vi "Actor Core.vi"(8 "error in":errorcluster, 11 "SensorCharm in":refnum<class "TimerSensorCharm.lvclass">) -> (0 "error out":errorcluster, 3 "Actor out":refnum<class "Actor.lvclass">)   [LabVIEW 2012, in "TimerSensor.lvlib" / "TimerSensorCharm.lvclass"]
doc: "(<B>Filename</B>: Actor Framework.lvlib:Actor.lvclass:Actor Core.vi)\n\nReceives messages to the actor, reacts to them, and initiates any error handling that may shut the actor down.\n\nDescendant classes may override this VI to append parallel tasks for the actor to complete while it handles messages. Overrides use the Call Parent Method node."
uses:
  TimerSensorCharm.lvclass
  <vilib>/ActorFramework/Actor/Actor.lvclass
  TimerView Sensor/Timer Direction.ctl
  Sensor Definition/SensorCharm.lvclass
  TimerSensorConfig.lvclass
  <vilib>/ActorFramework/Actor/Actor.lvclass/Actor.ctl
  <vilib>/ActorFramework/Message Enqueuer/Message Enqueuer.lvclass/Message Enqueuer.ctl
  Win8uiFramework/ViewableActor.lvclass/ViewableActor.ctl
  Sensor Definition/SensorCharm.lvclass/SensorCharm.ctl
  Sensor Definition/SensorInfo.lvclass/SensorInfo.ctl
  TimerSensorConfig.lvclass/TimerSensorConfig.ctl
  Sensor Messages/Update Sensor Info and Re-broadcast Msg/Update Sensor Info and Re-broadcast Msg.lvclass/Update Sensor Info and Re-broadcast Msg.ctl
  TimerView Sensor/Write Target Time.vi
  TimerView Sensor/Write Timer Direction.vi
  Sensor Definition/SensorInfo/Write Name.vi
  Sensor Definition/Write Description.vi
  Sensor Definition/SensorInfo/Write Config.vi
  Sensor Definition/SensorInfo/Write Sample Time.vi
  Win8uiFramework/Read Stop Event.vi
  Sensor Definition/SensorCharm/Read SensorInfo.vi
  Sensor Definition/SensorInfo/Read Name.vi
  Sensor Definition/SensorInfo/Read Description.vi
  Sensor Definition/Read Config.vi
  Sensor Definition/SensorInfo/Read Sample Time.vi
  TimerSensorConfig/Read Target Time.vi
  TimerSensorConfig/Read Timer Direction.vi
  <vilib>/ActorFramework/Message Enqueuer/Init from Existing Queue.vi
  <vilib>/ActorFramework/Message Enqueuer/Enqueue.vi
  <vilib>/ActorFramework/Message Priority Queue/Priority Enqueue.vi
  <vilib>/ActorFramework/Message Enqueuer/Message Enqueuer.lvclass
  Sensor Definition/SensorInfo.lvclass
  Sensor Definition/SensorConfig.lvclass
  Sensor Messages/Update Sensor Info and Re-broadcast Msg/Update Sensor Info and Re-broadcast Msg.lvclass
  Win8uiFramework/ViewableActor.lvclass
  TimerSensor.lvlib
panel:
  in  "Timer Direction":u16(ring) items=["Up", "Down"]
  in  "Timer Direction Enum":T1
  in  "Target Time":timestamp
  in  "Name":string="Name"
  in  "Sample Period (s)":dbl=1.0
  in  "Description":string="Description of what and/or where this sensor is."
  out "Title":string="Settings"
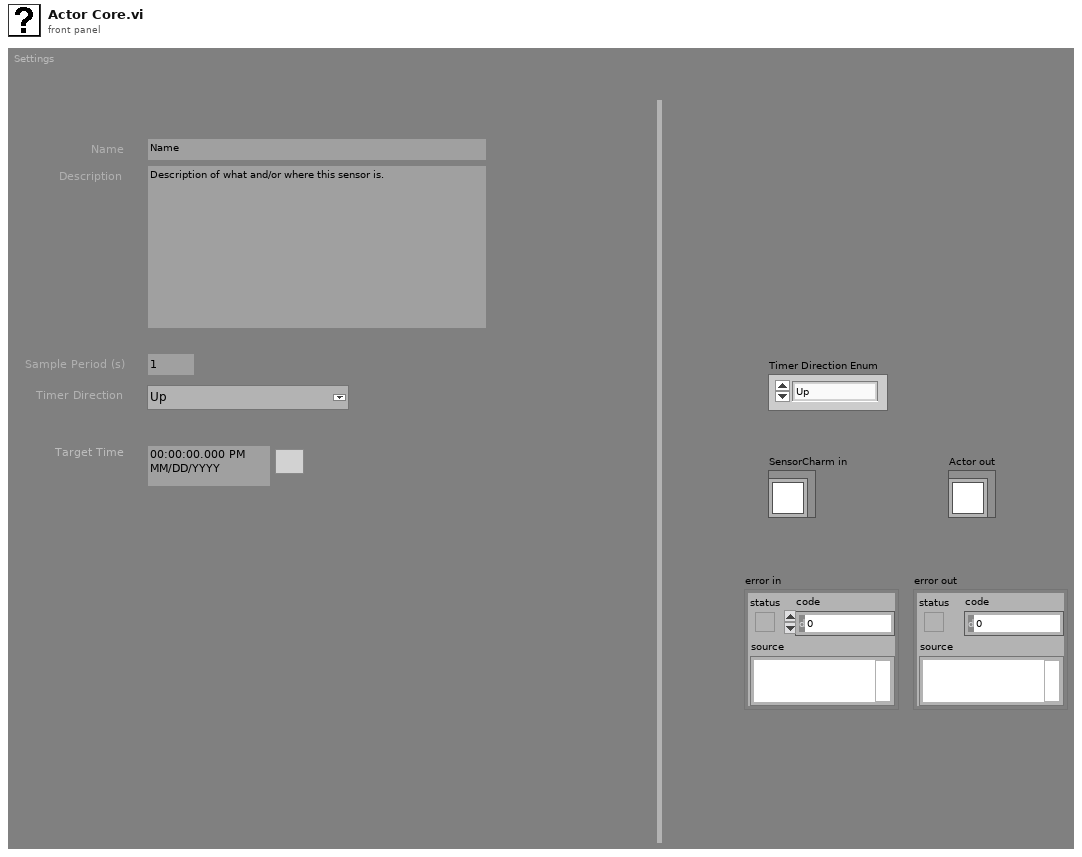
[diagram p1: front panel]
types:
  T1 = typedef "TimerSensor.lvlib/Timer Direction.ctl" = enum16{"Up", "Down"}
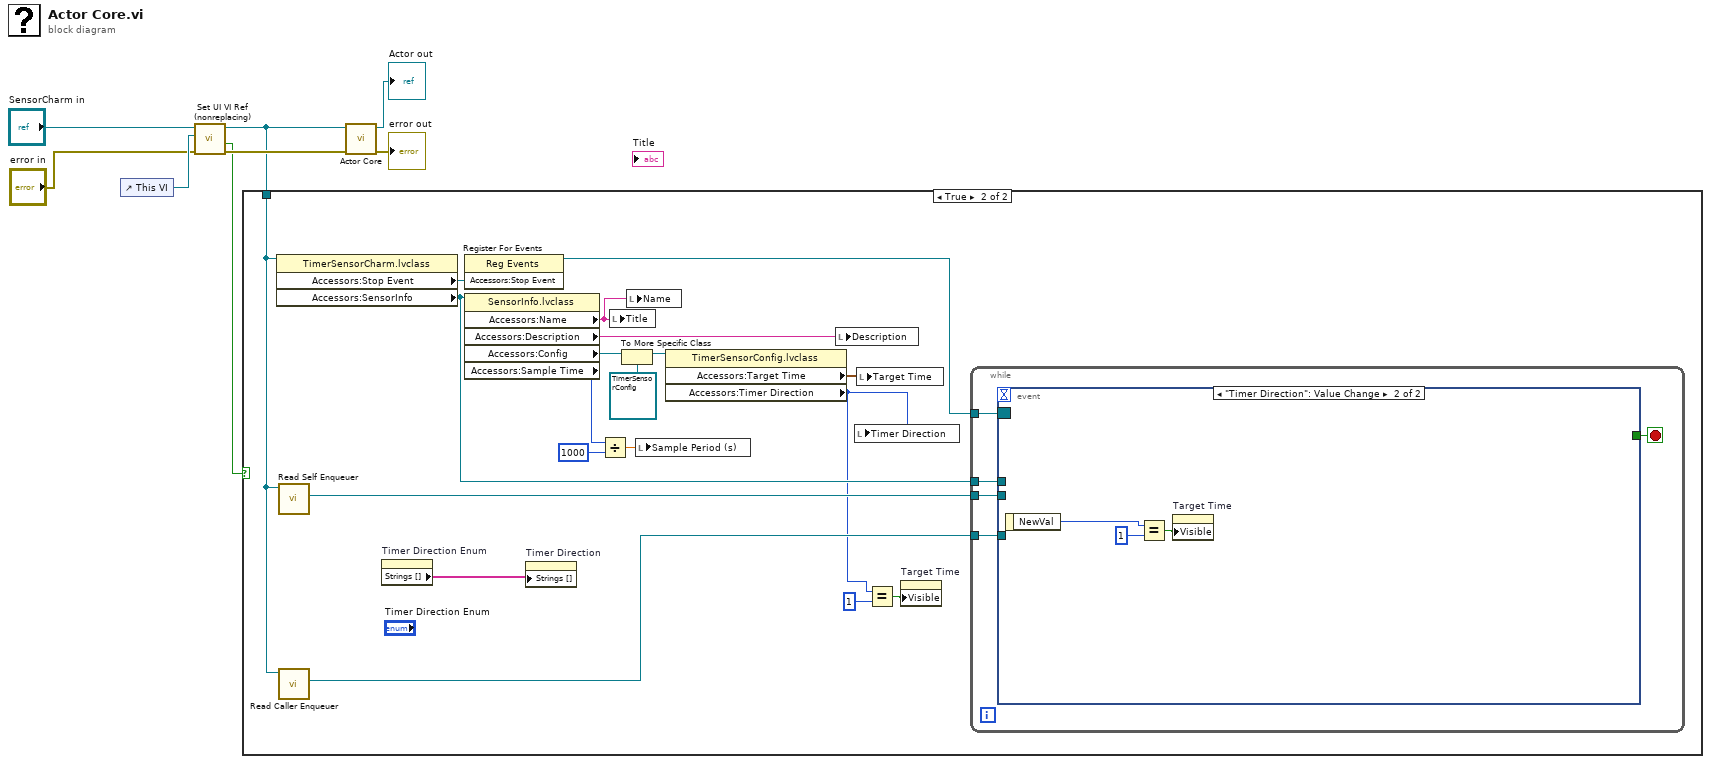
[diagram p0: block diagram]
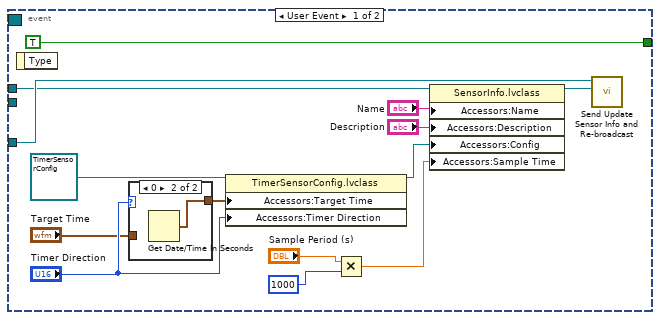
[diagram p3: hidden frame]
diagram:
  n1 = control-ref of="This VI"() -> (w6:refnum<vi>)
  n2 = call "Set UI VI Ref (nonreplacing).vi"("error in (no error)"="error in", "UI VI Ref"=w6, "ViewableActor in"="SensorCharm in") -> ("error out"=w3:errorcluster, "Top Level UI?"=w2:bool, "ViewableActor out"=w1:refnum<class "TimerSensorCharm.lvclass">)  [unwired: 6 in]
  n3 = case shown="True" w2 {
    tunnel: w1 -> [_ w24]
    frame False {
    }
    frame True {
      n4 = property class="TimerSensorCharm.lvclass"(reference=w24) -> ("Accessors:Stop Event"=w27:refnum<user-event>, "Accessors:SensorInfo"=w20:refnum<class "SensorInfo.lvclass">)  [unwired: 1 in, 2 out]
      n5 = call <vilib>:"Read Self Enqueuer.vi"("Actor"=w24) -> ("Self Enqueuer"=w25:refnum<class "Message Enqueuer.lvclass">)  [unwired: 10 in]
      n6 = call <vilib>:"Read Caller Enqueuer.vi"("Actor"=w24) -> ("Caller Enqueuer"=w23:refnum<class "Message Enqueuer.lvclass">)  [unwired: 10 in]
      n7 = property on="Timer Direction Enum" class="Enum (strict)"() -> ("Strings []"=w12:string[])  [unwired: 2 in, 2 out]
      n8 = register-events(w27) -> (reference out=w26:refnum<event-registration>)  [unwired: 2 in, 1 out]
      n9 = property class="SensorInfo.lvclass"(reference=w20) -> ("Accessors:Name"=w22:string, "Accessors:Description"=w21:string, "Accessors:Config"=w19:refnum<class "SensorConfig.lvclass">, "Accessors:Sample Time"=w15:i32)  [unwired: 1 in, 2 out]
      n10 = property on="Timer Direction" class="Ring (strict)"("Strings []"=w12) -> ()  [unwired: 2 in, 2 out]
      n11 = Divide(x=w15, y=1000) -> (x/y=w13:dbl)
      n12 = local write "Title"(w22) -> ()
      n13 = To More Specific Class(target class=refnum<class "TimerSensorConfig.lvclass"> refnum ("TimerSensor.lvlib:TimerSensorConfig.lvclass"), reference=w19) -> (specific class reference=w17:refnum<class "TimerSensorConfig.lvclass">)  [unwired: 1 in, 1 out]
      n14 = local write "Name"(w22) -> ()
      n15 = local write "Sample Period (s)"(w13) -> ()
      n16 = property class="TimerSensorConfig.lvclass"(reference=w17) -> ("Accessors:Target Time"=w16:timestamp, "Accessors:Timer Direction"=w9:T1)  [unwired: 1 in, 2 out]
      n17 = local write "Description"(w21) -> ()
      n18 = local write "Timer Direction"(w9) -> ()
      n19 = local write "Target Time"(w16) -> ()
      n20 = Equal?(x=w9, y=u16 1) -> (x = y?=w10:bool)
      n21 = property on="Target Time" class="AbsTime (strict)"("Visible"=w10) -> ()  [unwired: 2 in, 2 out]
      n22 = while {
        tunnel: w26 -> [w32]
        tunnel: w25 -> [w30]
        tunnel: w23 -> [w29]
        tunnel: w20 -> [w28]
        stop <- w31 stop-if-true
        n23 = event shown="[1] \"Timer Direction\": Value Change" {
          selector: w32 -> [_ _]
          dyn-events: _ -> [_ _]
          timeout: _ -> [_ _]
          tunnel: [TRUE _] -> w31
          tunnel: w30 -> [_ _]
          tunnel: w29 -> [w45 _]
          tunnel: w28 -> [w44 _]
          event User Event {
            n24 = event-data() -> ()  [unwired: 1 in, 1 out]
            n25 = case shown="0" "Timer Direction" {
              tunnel: "Target Time" -> [w47 _]
              tunnel: [w47 w48] -> w33
              frame 1, Default {
              }
              frame 0 {
                n26 = Get Date/Time In Seconds() -> (seconds since 1Jan1904=w48:timestamp)
              }
            }
            n27 = property class="TimerSensorConfig.lvclass"(reference=refnum<class "TimerSensorConfig.lvclass"> refnum ("TimerSensor.lvlib:TimerSensorConfig.lvclass"), "Accessors:Target Time"=w33, "Accessors:Timer Direction"="Timer Direction") -> (reference out=w39:refnum<class "TimerSensorConfig.lvclass">)  [unwired: 1 in, 1 out]
            n28 = Multiply(x="Sample Period (s)", y=1000) -> (x*y=w37:dbl)
            n29 = property class="SensorInfo.lvclass"(reference=w44, "Accessors:Name"="Name", "Accessors:Description"="Description", "Accessors:Config"=w39, "Accessors:Sample Time"=w37) -> (reference out=w41:refnum<class "SensorInfo.lvclass">)  [unwired: 1 in, 1 out]
            n30 = call "Send Update Sensor Info and Re-broadcast.vi"("SensorInfo"=w41, "Message Enqueuer"=w45) -> ()  [unwired: 8 in, 2 out]
          }
          event "Timer Direction": Value Change {
            n31 = event-data() -> ("NewVal"=w51:u16)  [unwired: 1 in]
            n32 = Equal?(x=w51, y=u16 1) -> (x = y?=w50:bool)
            n33 = property on="Target Time" class="AbsTime (strict)"("Visible"=w50) -> ()  [unwired: 2 in, 2 out]
          }
        }
      }
    }
  }
  n34 = call-parent "Actor Core.vi"("error in"=w3, "SensorCharm in"=w1) -> ("error out"=→"error out":errorcluster, "Actor out"=→"Actor out":refnum<class "Actor.lvclass">)  [unwired: 8 in]
